vi "TCP-Disconnect.vi"(0 "connection ID":refnum<k5>, 9 "timeout (ms)":i32=5000, 11 "error in (no error)":errorcluster) -> (15 "error out":errorcluster)   [LabVIEW 2020]
panel:
  out "result":i32
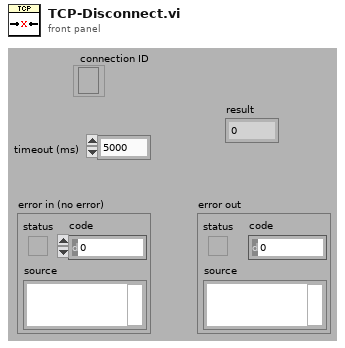
[diagram p1: front panel]
types:
  T1 = enum16{"Standard", "Buffered", "CRLF", "Immediate"}
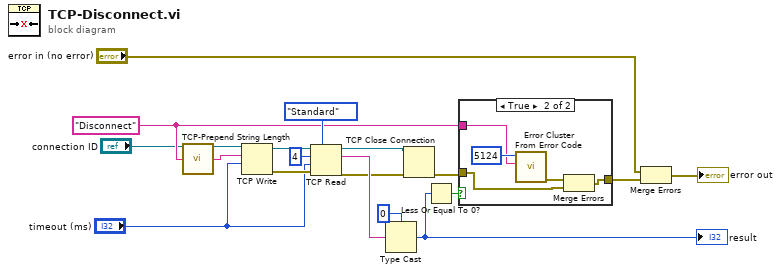
[diagram p0: block diagram]
diagram:
  w7 = "Disconnect" ("Command")
  n1 = call "TCP-Prepend String Length.vi"("Command"=w7) -> ("String"=w6:string)  [unwired: 4 in]
  n2 = TCP Write(connection ID="connection ID", data in=w6, 9:"timeout (ms)") -> (connection ID out=w18:refnum<k5>, error out=w9:errorcluster)  [unwired: 1 in, 1 out]
  n3 = TCP Read(connection ID=w18, bytes to read=4, error in (no error)=w9, 7:T1."Standard" ("mode (standard)"), 9:"timeout (ms)") -> (connection ID out=w2:refnum<k5>, data out=w17:string, error out=w1:errorcluster)
  n4 = Type Cast(type=0, x=w17) -> (*(type *) &x=w8:i32)
  "result" <- w8
  n5 = TCP Close Connection(connection ID=w2, error in (no error)=w1) -> (error out=w3:errorcluster)  [unwired: 1 in, 1 out]
  n6 = Less Or Equal To 0?(x=w8) -> (x <= 0?=w15:bool)
  n7 = case shown="True" w15 {
    tunnel: [w19 w21] -> w14
    tunnel: w3 -> [w19 w20]
    tunnel: w7 -> [_ w22]
    frame False {
    }
    frame True {
      n8 = call <vilib>:"Error Cluster From Error Code.vi"("error message (\"\")"=w22, "error code (0)"=5124) -> ("error out"=w24:errorcluster)  [unwired: 7 in]
      n9 = Merge Errors(w24, w20) -> (w21:errorcluster)
    }
  }
  n10 = Merge Errors("error in (no error)", w14) -> (→"error out":errorcluster)
